vi "Ports.vi"(0 "Test":string, 1 "Reserved array Input":string[](array[string])) -> (2 "Result Input":string[](array[string]), 3 "Ports counter":i32, 4 "Sizes":i32[](array[numeric]))   [LabVIEW 2012]
panel:
  out "before substring":string
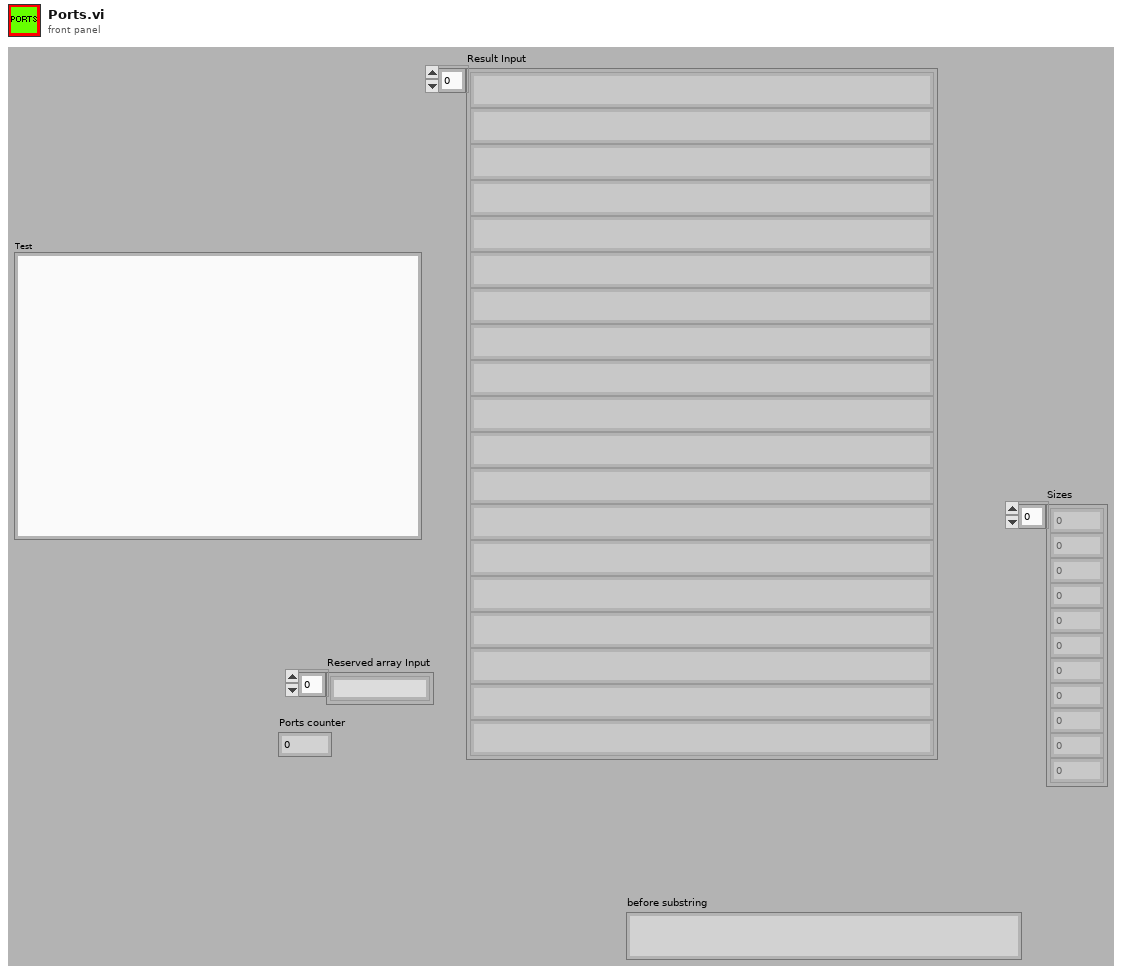
[diagram p1: front panel]
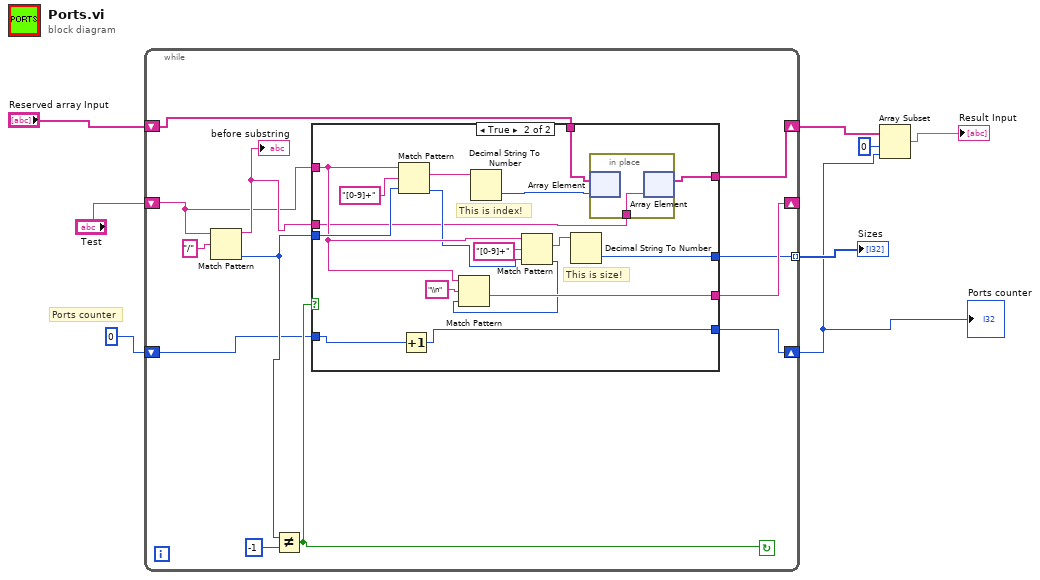
[diagram p0: block diagram]
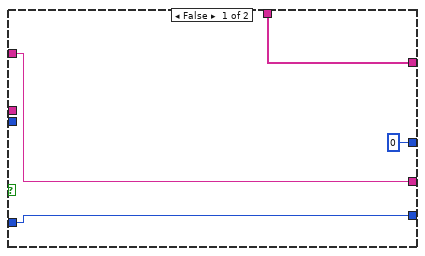
[diagram p2: hidden frame]
diagram:
  # "Ports counter"
  n1 = while {
    shift-right: [w15] -> w4
    shift-left: "Reserved array Input" -> [w17]
    shift-right: [w12] -> w2
    shift-left: 0 ("offset past match") -> [w13]
    shift-right: [w11] -> _
    shift-left: "Test" -> [w10]
    tunnel: [w9] -> w5 mode=indexing
    stop <- w14 continue-if-true
    n2 = Match Pattern(string=w10, regular expression="/" ("search string")) -> (before substring=w16:string, offset past match=w18:i32)  [unwired: 1 in, 2 out]
    "before substring" <- w16
    n3 = Not Equal?(x=w18, y=-1) -> (x != y?=w14:bool)
    n4 = case shown="True" w14 {
      tunnel: w10 -> [w22 w34]
      tunnel: w18 -> [_ w41]
      tunnel: w17 -> [w24 w28]
      tunnel: w16 -> [_ w26]
      tunnel: [w24 w25] -> w15
      tunnel: w13 -> [w23 w37]
      tunnel: [w23 w36] -> w12
      tunnel: [w22 w35] -> w11
      tunnel: [0 w29] -> w9
      frame False {
      }
      frame True {
        # "This is size!"
        # "This is index!"
        n5 = Match Pattern(string=w34, regular expression="[0-9]+", offset (0)=w41) -> (match substring=w39:string, offset past match=w32:i32)  [unwired: 2 out]
        n6 = Increment(x=w37) -> (x+1=w36:i32)
        n7 = Decimal String To Number(string=w39) -> (number=w27:i32)  [unwired: 2 in, 1 out]
        n8 = Match Pattern(string=w34, regular expression="[0-9]+", offset (0)=w32) -> (match substring=w31:string, offset past match=w30:i32)  [unwired: 2 out]
        n9 = Match Pattern(string=w34, regular expression="\\n" ("search string"), offset (0)=w30) -> (after substring=w35:string)  [unwired: 3 out]
        n10 = Decimal String To Number(string=w31) -> (number=w29:i32)  [unwired: 2 in, 1 out]
        n11 = in-place {
          in-place-border: w26 -> [w42]
          n12 = in-place-array #1(w28, w27) -> ()  [unwired: 1 out]
          n13 = in-place-array #1(w42) -> (w25:string[])  [unwired: 1 out]
        }
      }
    }
  }
  "Ports counter" <- w2
  "Sizes" <- w5
  n14 = Array Subset(array=w4, index=0, length=w2) -> (→"Result Input":string[])
